vi "Write Sheet2 Data.vi"(8 "Cal Point":i32, 9 "Dev Table 1":string[][](array[string]), 10 "Actual Table 1":string[][](array[string]), 11 "Cal Path":path) -> ()   [LabVIEW 2013]
uses:
  Type Defs/Excel Driver Operator Type Def.ctl
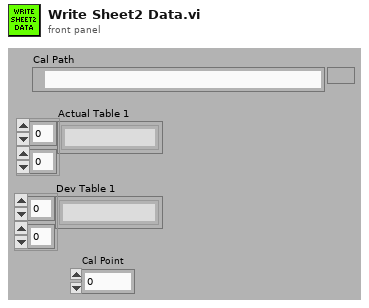
[diagram p1: front panel]
types:
  T1 = typedef "Excel Driver Operator Type Def.ctl" = enum16{"Open", "Close", "Search for String", "GetUsedRange", "Read Range", "Read Cell", "Set Range", "Set Cell"}
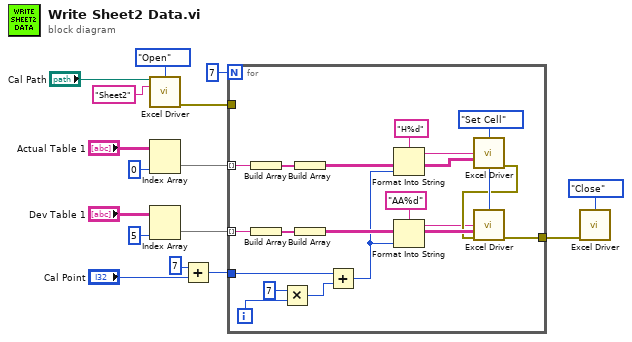
[diagram p0: block diagram]
diagram:
  n1 = call "Excel Driver.vi"("Filename of Workbook"="Cal Path", "Operator"=Excel_Driver_Operator_Type_Def."Open", "WorkSheet Name"="Sheet2") -> ("error out"=w7:errorcluster)  [unwired: 10 in, 2 out]
  n2 = Index Array(array="Actual Table 1", index (col)=0 ("disabled index (col)")) -> (element=w9:string[])  [unwired: 1 in]
  n3 = Index Array(array="Dev Table 1", index (col)=5 ("disabled index (col)")) -> (element=w8:string[])  [unwired: 1 in]
  n4 = Add(x=7 ("disabled index (col)"), y="Cal Point") -> (x+y=w2:i32)
  n5 = for {
    N: 7 -> [_]
    tunnel: w9 -> [w32] mode=indexing
    tunnel: w8 -> [w28] mode=indexing
    tunnel: w2 -> [w17]
    tunnel: w7 -> [_]
    tunnel: [w24] -> w5
    i -> [w19]
    w26 = Excel_Driver_Operator_Type_Def."Set Cell" ("Operator")
    n6 = Build Array(w32) -> (w31:string[])
    n7 = Build Array(w28) -> (w29:string[])
    n8 = Multiply(x=7 ("disabled index (col)"), y=w19) -> (x*y=w21:i32)
    n9 = Build Array(w31) -> (w30:string[][])
    n10 = Build Array(w29) -> (w27:string[][])
    n11 = Add(x=w17, y=w21) -> (x+y=w20:i32)
    n12 = Format Into String(format string="H%d", w20) -> (resulting string=w23:string)  [unwired: 2 in, 1 out]
    n13 = Format Into String(format string="AA%d", w20) -> (resulting string=w22:string)  [unwired: 2 in, 1 out]
    n14 = call "Excel Driver.vi"("Operator"=w26, "Range String\n(Or Search String)"=w23, "Cell Values INPUT"=w30) -> ("error out"=w25:errorcluster)  [unwired: 10 in, 2 out]
    n15 = call "Excel Driver.vi"("Operator"=w26, "Range String\n(Or Search String)"=w22, "Cell Values INPUT"=w27, "error in (no error)"=w25) -> ("error out"=w24:errorcluster)  [unwired: 9 in, 2 out]
  }
  n16 = call "Excel Driver.vi"("Operator"=Excel_Driver_Operator_Type_Def."Close", "error in (no error)"=w5) -> ()  [unwired: 11 in, 3 out]
